vi "PH_VacuumControl.ProcEvents.vi"(0 "i ref in":refnum<vi>, 5 "error in":errorcluster) -> (14 "i ref out":refnum<vi>, 19 "error out":errorcluster)   [LabVIEW 2014, in "PH_VacuumControl.lvlib"]
doc: "This method is used to define the events the object will listen to. Add your own events here."
uses:
  PH_VacuumControl.lvlib
  CS_Core/BaseProcess/BaseProcess.event definition.ctl
  CS_Core/CAEObj/CAEObj.event definition.ctl
  CS_Core/BaseProcess/BaseProcess.descriptor string definition.ctl
  CS_Core/BaseProcess/BaseProcess.lvlib
  CS_Core/CAEObj/CAEObj.lvlib
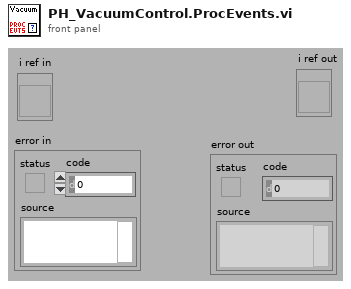
[diagram p1: front panel]
types:
  T1 = typedef "BaseProcess.lvlib/BaseProcess.event definition.ctl" = cluster{"CAEEvtDef":T2, "Data Descriptor":T3}
  T2 = typedef "CAEObj.lvlib/CAEObj.event definition.ctl" = cluster{"URL":string, "enable":bool, "ignoreResID":bool}
  T3 = typedef "BaseProcess.lvlib/BaseProcess.descriptor string definition.ctl" = string
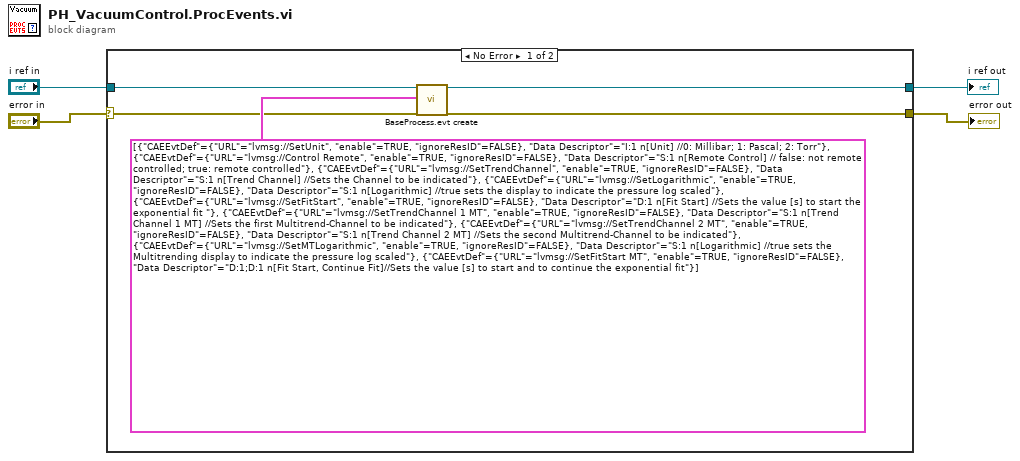
[diagram p0: block diagram]
diagram:
  n1 = case shown="No Error" "error in" {
    selector: "error in" -> [w5 w10]
    tunnel: "i ref in" -> [w9 w11]
    tunnel: [w7 w10] -> w3
    tunnel: [w6 w11] -> w2
    frame No Error {
      n2 = call "BaseProcess.evt create.vi"("i ref in"=w9, "newEvents"=T1[] [{"CAEEvtDef"={"URL"="lvmsg://SetUnit", "enable"=TRUE, "ignoreResID"=FALSE}, "Data Descriptor"="I:1 n[Unit] //0: Millibar; 1: Pascal; 2: Torr"}, {"CAEEvtDef"={"URL"="lvmsg://Control Remote", "enable"=TRUE, "ignoreResID"=FALSE}, "Data Descriptor"="S:1 n[Remote Control] // false: not remote controlled; true: remote controlled"}, {"CAEEvtDef"={"URL"="lvmsg://SetTrendChannel", "enable"=TRUE, "ignoreResID"=FALSE}, "Data Descriptor"="S:1 n[Trend Channel] //Sets the Channel to be indicated"}, {"CAEEvtDef"={"URL"="lvmsg://SetLogarithmic", "enable"=TRUE, "ignoreResID"=FALSE}, "Data Descriptor"="S:1 n[Logarithmic] //true sets the display to indicate the pressure log scaled"}, {"CAEEvtDef"={"URL"="lvmsg://SetFitStart", "enable"=TRUE, "ignoreResID"=FALSE}, "Data Descriptor"="D:1 n[Fit Start] //Sets the value [s] to start the exponential fit "}, {"CAEEvtDef"={"URL"="lvmsg://SetTrendChannel 1 MT", "enable"=TRUE, "ignoreResID"=FALSE}, "Data Descriptor"="S:1 n[Trend Channel 1 MT] //Sets the first Multitrend-Channel to be indicated"}, {"CAEEvtDef"={"URL"="lvmsg://SetTrendChannel 2 MT", "enable"=TRUE, "ignoreResID"=FALSE}, "Data Descriptor"="S:1 n[Trend Channel 2 MT] //Sets the second Multitrend-Channel to be indicated"}, {"CAEEvtDef"={"URL"="lvmsg://SetMTLogarithmic", "enable"=TRUE, "ignoreResID"=FALSE}, "Data Descriptor"="S:1 n[Logarithmic] //true sets the Multitrending display to indicate the pressure log scaled"}, {"CAEEvtDef"={"URL"="lvmsg://SetFitStart MT", "enable"=TRUE, "ignoreResID"=FALSE}, "Data Descriptor"="D:1;D:1 n[Fit Start, Continue Fit]//Sets the value [s] to start and to continue the exponential fit"}] ("new events"), "error in (no error)"=w5) -> ("i ref out"=w6:refnum<vi>, "error out"=w7:errorcluster)  [unwired: 13 in, 2 out]
    }
    frame Error {
    }
  }
  "i ref out" <- w2
  "error out" <- w3
